vi "ReadContinuous.vi"() -> ()   [LabVIEW 2016]
doc: "testing detection of release and squeeze in a number of ways"
uses:
  UsbScShdlc_Sensirion/control/modeReadWrite_UsbScShdlc_Sensirion.ctl
  UsbScShdlc_Sensirion/control/SensorVoltage_UsbScShdlc_Sensirion.ctl
  UsbScShdlc_Sensirion/control/SensorType_UsbScShdlc_Sensirion.ctl
  <vilib>/Analysis/NI_AALPro.lvlib
  <vilib>/Analysis/NI_AALBase.lvlib
  <vilib>/addons/Wavelet Analysis/application.llb/WA Detrend (Array).vi
  <vilib>/Analysis/3filter.llb/Equi-Ripple HighPass (DBL).vi
  UsbScShdlc_Sensirion/control/InterlacedDataSF06_UsbScShdlc_Sensirion.ctl
panel:
  out "integral 3":dbl[](graph) caption="Waveform Graph"
  out "integral 2":dbl[](graph) caption="Waveform Graph"
  out "x/y":dbl[](array[numeric])
  in  "zero":dbl=0.05 step=0.001 format="%#_13g"
  out "integral":dbl[](graph) caption="Waveform Graph"
  out "NumberOfPackagesRemainingInBuffer":u16
  out "NumberOfMeasuredPackagesLost":u32
  out "TotalOfLostPackages\n(at measurement end)":u32
  out "listNumberOfMeasuredPackagesLost":u32[](array[numeric])
  out "Data temperature":dbl[](graph) caption="Waveform Graph"
  in  "ScaleFactor Temp":u16=200 caption="Measurement interval [ms]"
  in  "ScaleFactor flow/dp":u16=60 caption="Measurement interval [ms]"
  in  "stop":bool
  out "readInterlacedDataSF06":T1
  in  "AdditionalParameter\n(for used command)":u8[](array[numeric]) format="%.0x"
  in  "Command":u16=13827 caption="Measurement interval [ms]" format="%.0x"
  out "FoundI2cAddresses":u8[](array[numeric]) caption="Rx data" format="%02x"
  out "Data flow/dp":dbl[](graph) caption="Waveform Graph"
  out "NumberOfMeasurements":u16
  in  "Measurement interval [ms]":u16=1
  in  "address (USB SensorCable)":u8 caption="address" format="%02x"
  in  "COM port":refnum<visa-resource-name>
  in  "error in (no error)":errorcluster
  out "error out":errorcluster
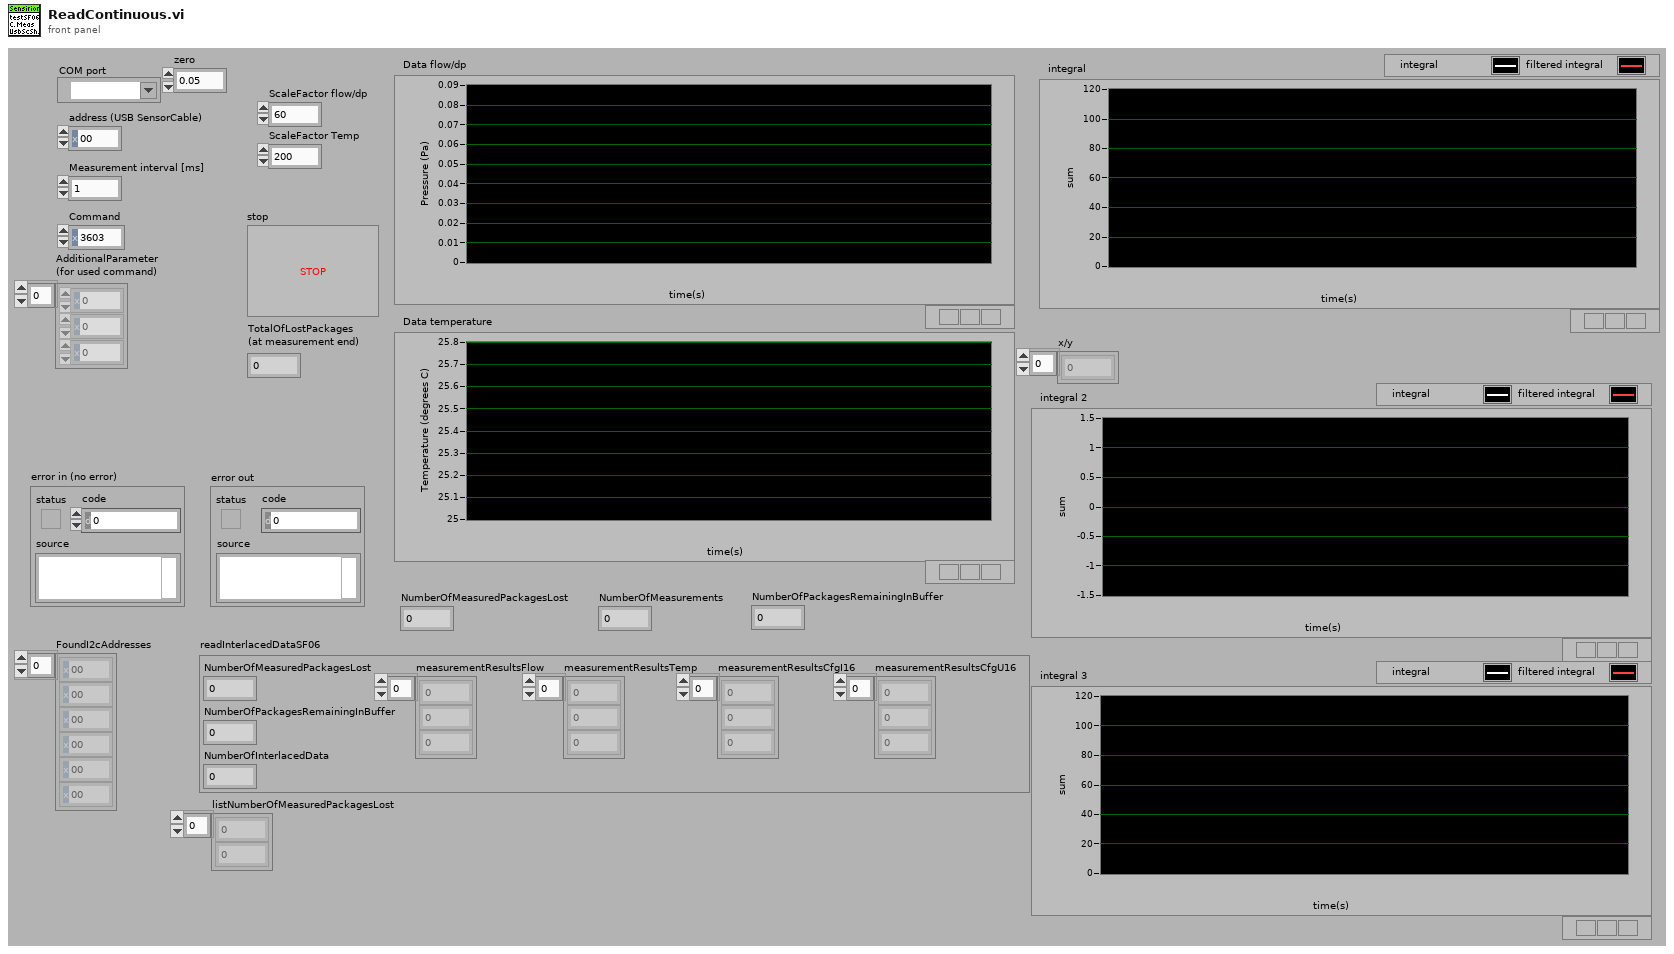
[diagram p1: front panel]
types:
  T1 = typedef "InterlacedDataSF06_UsbScShdlc_Sensirion.ctl" = cluster{"NumberOfMeasuredPackagesLost":u32, "NumberOfPackagesRemainingInBuffer":u16, "NumberOfInterlacedData":u16, "measurementResultsFlow":i16[], "measurementResultsTemp":i16[], "measurementResultsCfgI16":i16[], "measurementResultsCfgU16":u16[]}
  T2 = typedef "SensorType_UsbScShdlc_Sensirion.ctl" = enum16{"SF04 Flow Sensor", "Humidity Sensor", "SF05 Flow Sensor", "SF06 Flow Sensor"}
  T3 = typedef "SensorVoltage_UsbScShdlc_Sensirion.ctl" = enum16{"3.3V", "5.0V"}
  T4 = typedef "modeReadWrite_UsbScShdlc_Sensirion.ctl" = bool
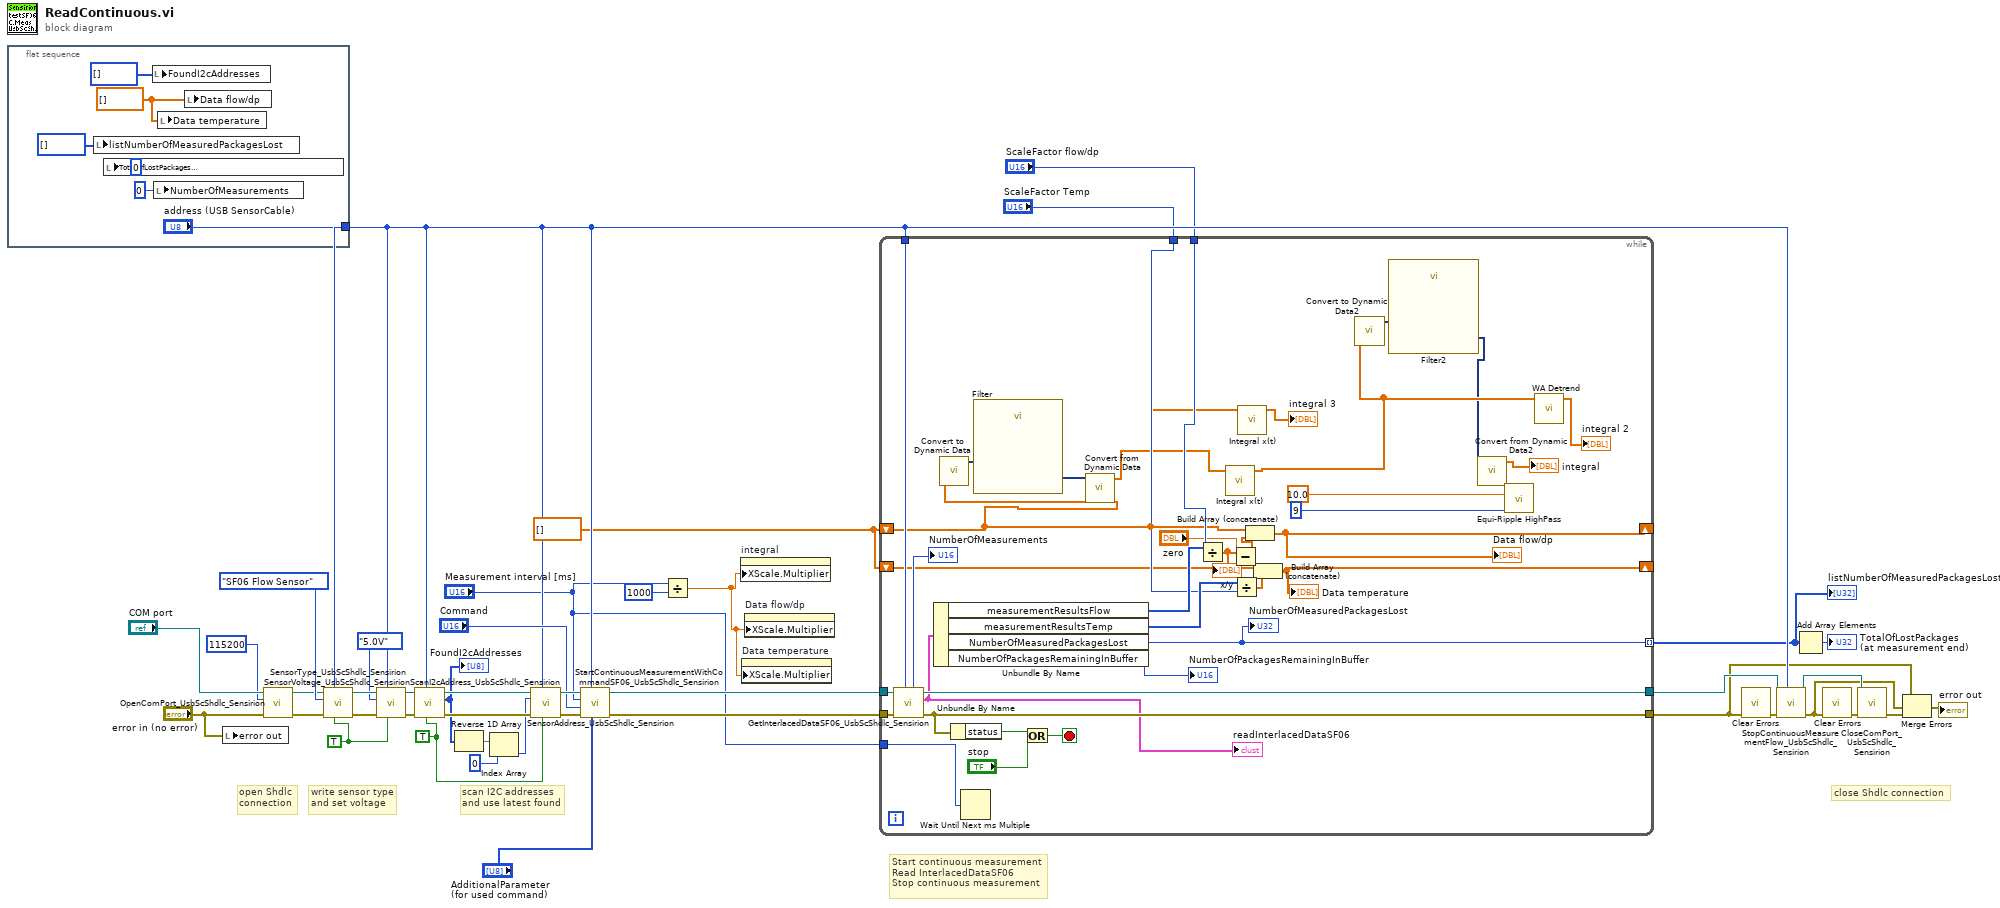
[diagram p0: block diagram]
diagram:
  w14 = dbl[] []
  w31 = TRUE ("range")
  w34 = T4 TRUE ("mode")
  # "scan I2C addresses \nand use latest found"
  # "close Shdlc connection"
  # "Start continuous measurement\nRead InterlacedDataSF06\nStop continuous measurement"
  # "write sensor type\nand set voltage"
  # "open Shdlc\nconnection"
  n1 = flat-sequence {
    tunnel: ["address (USB SensorCable)"] -> w19
    frame #0 {
      w46 = dbl[] [] ("Data flow/dp")
      n2 = local write "listNumberOfMeasuredPackagesLost"(u32[] [] ("listNumberOfMeasuredPackagesLost")) -> ()
      n3 = local write "TotalOfLostPackages\n(at measurement end)"(u32 0 ("TotalOfLostPackages")) -> ()
      n4 = local write "FoundI2cAddresses"(u8[] [] ("FoundI2cAddresses")) -> ()
      n5 = local write "NumberOfMeasurements"(u16 0 ("NumberOfMeasurements")) -> ()
      n6 = local write "Data temperature"(w46) -> ()
      n7 = local write "Data flow/dp"(w46) -> ()
    }
  }
  n8 = local write "error out"("error in (no error)") -> ()
  n9 = call "OpenComPort_UsbScShdlc_Sensirion.vi"("error in (no error)"="error in (no error)", "baud rate (115200)"=u32 115200, "COM port"="COM port") -> ("error out"=w35:errorcluster, "COM port out"=w36:refnum<visa-resource-name>)  [unwired: 7 in]
  n10 = call "SensorType_UsbScShdlc_Sensirion.vi"("mode"=w34, "address"=w19, "error in (no error)"=w35, "SensorType"=SensorType_UsbScShdlc_Sensirion."SF06 Flow Sensor", "COM port"=w36) -> ("error out"=w39:errorcluster, "COM port out"=w38:refnum<visa-resource-name>)  [unwired: 4 in, 1 out]
  n11 = call "SensorVoltage_UsbScShdlc_Sensirion.vi"("mode"=w34, "address"=w19, "error in (no error)"=w39, "SensorVoltage"=SensorVoltage_UsbScShdlc_Sensirion."5.0V", "COM port"=w38) -> ("error out"=w26:errorcluster, "COM port out"=w25:refnum<visa-resource-name>)  [unwired: 4 in, 1 out]
  n12 = call "ScanI2cAddress_UsbScShdlc_Sensirion.vi"("range"=w31, "address"=w19, "error in (no error)"=w26, "COM port"=w25) -> ("error out"=w33:errorcluster, "FoundI2cAddresses"=w30:u8[], "COM port out"=w32:refnum<visa-resource-name>)  [unwired: 5 in]
  "FoundI2cAddresses" <- w30
  n13 = Reverse 1D Array(array=w30) -> (reversed array=w29:u8[])
  n14 = Index Array(array=w29, index=0) -> (element=w27:u8)
  n15 = call "SensorAddress_UsbScShdlc_Sensirion.vi"("mode"=w31, "address"=w19, "error in (no error)"=w33, "SensorAddress"=w27, "COM port"=w32) -> ("error out"=w23:errorcluster, "COM port out"=w24:refnum<visa-resource-name>)  [unwired: 4 in, 1 out]
  n16 = call "StartContinuousMeasurementWithCommandSF06_UsbScShdlc_Sensirion.vi"("AdditionalParameter"="AdditionalParameter\n(for used command)", "address"=w19, "error in (no error)"=w23, "Command"="Command", "Measurement interval [ms]"="Measurement interval [ms]", "COM port"=w24) -> ("error out"=w10:errorcluster, "COM port out"=w20:refnum<visa-resource-name>)  [unwired: 4 in]
  n17 = Divide(x="Measurement interval [ms]", y=u16 1000) -> (x/y=w2:dbl)
  n18 = property on="integral" class="WFGraph (strict)"("XScale.Multiplier"=w2) -> ()  [unwired: 2 in, 2 out]
  n19 = property on="Data temperature" class="WFGraph (strict)"("XScale.Multiplier"=w2) -> ()  [unwired: 2 in, 2 out]
  n20 = property on="Data flow/dp" class="WFGraph (strict)"("XScale.Multiplier"=w2) -> ()  [unwired: 2 in, 2 out]
  n21 = while {
    tunnel: w10 -> [w84]
    tunnel: w20 -> [w83]
    tunnel: w19 -> [w82]
    tunnel: [w81] -> w7
    tunnel: [w80] -> w6
    tunnel: [w76] -> w12 mode=indexing
    shift-right: [w67] -> _
    shift-left: w14 -> [w51]
    tunnel: "ScaleFactor flow/dp" -> [w73]
    shift-right: [w66] -> _
    shift-left: w14 -> [w68]
    tunnel: "ScaleFactor Temp" -> [w70]
    tunnel: "Measurement interval [ms]" -> [w49]
    stop <- w77 stop-if-true
    n22 = call "GetInterlacedDataSF06_UsbScShdlc_Sensirion.vi"("address"=w82, "error in (no error)"=w84, "COM port"=w83) -> ("error out"=w80:errorcluster, "InterlacedDataSF06"=w65:T1, "COM port out"=w81:refnum<visa-resource-name>, "ReadDataSets"=→"NumberOfMeasurements":u16)  [unwired: 5 in]
    "readInterlacedDataSF06" <- w65
    n23 = Unbundle By Name(w65) -> ("measurementResultsFlow"=w75:i16[], "measurementResultsTemp"=w71:i16[], "NumberOfMeasuredPackagesLost"=w76:u32, "NumberOfPackagesRemainingInBuffer"=→"NumberOfPackagesRemainingInBuffer":u16)
    "NumberOfMeasuredPackagesLost" <- w76
    n24 = call "Convert to Dynamic Data"("Array"=w51) -> ("Dynamic Data Type"=w59:dynamicdata)  [unwired: 3 in]
    n25 = Unbundle By Name(w80) -> ("status"=w79:bool)
    n26 = Wait Until Next ms Multiple(millisecond multiple=w49) -> ()  [unwired: 1 out]
    n27 = call "Filter"("Signal"=w59) -> ("Filtered Signal"=w58:dynamicdata)  [unwired: 9 in, 1 out]
    n28 = Or(x=w79, y="stop") -> (x .or. y?=w77:bool)
    n29 = call "Convert from Dynamic Data"("Dynamic Data Type"=w58) -> ("Array"=w57:dbl[])  [unwired: 3 in]
    n30 = Divide(x=w75, y=w73) -> (x/y=w72:dbl[])
    "x/y" <- w72
    n31 = call <vilib>:"Integral x(t).vi"("X"=w57) -> ("Integral X"=w56:dbl[])  [unwired: 9 in, 1 out]
    n32 = Subtract(x=w72, y="zero") -> (x-y=w62:dbl[])
    n33 = Divide(x=w71, y=w70) -> (x/y=w69:dbl[])
    n34 = call <vilib>:"Integral x(t).vi"("X"=w51) -> ("Integral X"=→"integral 3":dbl[])  [unwired: 9 in, 1 out]
    n35 = Build Array (concatenate)(w51, w62) -> (w67:dbl[])
    "Data flow/dp" <- w67
    n36 = Build Array (concatenate)(w68, w69) -> (w66:dbl[])
    "Data temperature" <- w66
    n37 = call "Convert to Dynamic Data2"("Array"=w56) -> ("Dynamic Data Type"=w55:dynamicdata)  [unwired: 3 in]
    n38 = call "Filter2"("Signal"=w55) -> ("Filtered Signal"=w54:dynamicdata)  [unwired: 9 in, 1 out]
    n39 = call "Convert from Dynamic Data2"("Dynamic Data Type"=w54) -> ("Array"=→"integral":dbl[])  [unwired: 3 in]
    n40 = call-poly <vilib>:"Equi-Ripple HighPass.vi"("# of taps"=9, "sampling freq: fs"=10.0) -> ()  [unwired: 4 in, 2 out]
    n41 = call-poly <vilib>:"WA Detrend.vi"("signal"=w56) -> ("detrended signal"=→"integral 2":dbl[])  [unwired: 8 in, 2 out]
  }
  "listNumberOfMeasuredPackagesLost" <- w12
  n42 = call <vilib>:"Clear Errors.vi"("error in (no error)"=w6) -> ("error out"=w17:errorcluster)  [unwired: 5 in, 1 out]
  n43 = call "StopContinuousMeasurementFlow_UsbScShdlc_Sensirion.vi"("address"=w19, "error in (no error)"=w17, "COM port"=w7) -> ("error out"=w4:errorcluster, "COM port out"=w18:refnum<visa-resource-name>)  [unwired: 7 in]
  n44 = Add Array Elements(numeric array=w12) -> (sum=→"TotalOfLostPackages\n(at measurement end)":u32)
  n45 = call <vilib>:"Clear Errors.vi"("error in (no error)"=w4) -> ("error out"=w16:errorcluster)  [unwired: 5 in, 1 out]
  n46 = call "CloseComPort_UsbScShdlc_Sensirion.vi"("error in (no error)"=w16, "COM port"=w18) -> ("error out"=w5:errorcluster)  [unwired: 9 in]
  n47 = Merge Errors(w6, w4, w5) -> (→"error out":errorcluster)
